vi "Other Output Item UI Update.vi"(8 "error in (no error)":errorcluster, 10 "Other UI Elements":T1, 11 "Output":T2) -> (0 "error out":errorcluster)   [LabVIEW 2015, in "OutputUI.lvclass"]
uses:
  OutputUI.lvclass
  Step/STEP_OUTPUT.ctl
  Step/OUTPUT_DATA_TYPE.ctl
  OUTPUT_CHECK_TYPE.ctl
  Step/OUTPUT_VALUE_TYPE.ctl
  Step.lvclass
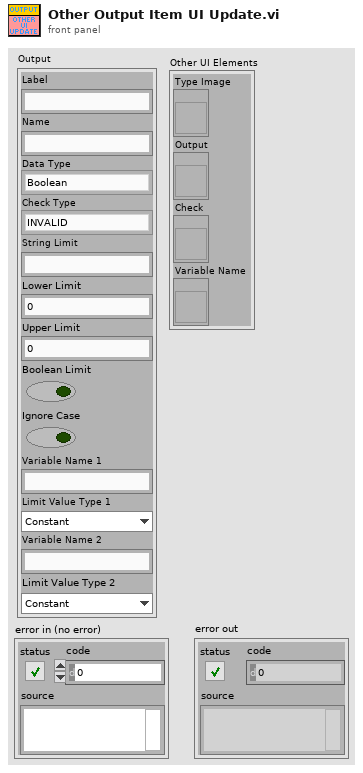
[diagram p1: front panel]
types:
  T1 = cluster{"Type Image":refnum<vi>, "Output":refnum<vi>, "Check":refnum<vi>, "Variable Name":refnum<vi>}
  T2 = typedef "Step.lvclass/STEP_OUTPUT.ctl" = cluster{"Label":string, "Name":string, "Data Type":T3, "Check Type":T4, "String Limit":string, "Lower Limit":dbl, "Upper Limit":dbl, "Boolean Limit":bool, "Ignore Case":bool, "Variable Name 1":string, "Limit Value Type 1":T5, "Variable Name 2":string, "Limit Value Type 2":T5}
  T3 = typedef "Step.lvclass/OUTPUT_DATA_TYPE.ctl" = enum16{"Boolean", "String", "Numeric", "Other"}
  T4 = typedef "Step.lvclass/OUTPUT_CHECK_TYPE.ctl" = enum16{"INVALID", "DO_NOT_CHECK", "RECORD", "VARIABLE", "EQUAL", "NOT_EQUAL", "STR_CONTAINS", "STR_START_WITH", "STR_END_WITH", "STR_REGEX_MATCH", "NUM_GT", "NUM_LT", "NUM_GE", "NUM_LE", "NUM_RANGE", "NUM_RANGE_BDY"}
  T5 = typedef "Step.lvclass/OUTPUT_VALUE_TYPE.ctl" = enum16{"Constant", "Variable"}
  T6 = enum8{"Enabled", "Disabled", "Disabled and Grayed Out"}
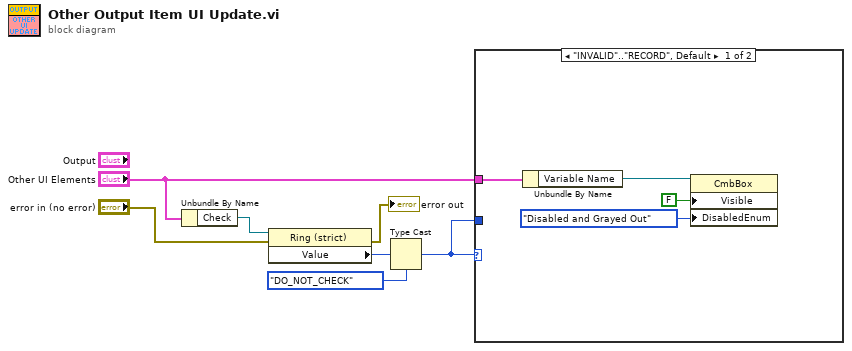
[diagram p0: block diagram]
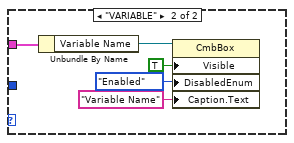
[diagram p2: hidden frame]
diagram:
  n1 = Unbundle By Name("Other UI Elements") -> ("Check"=w7:refnum<vi>)
  n2 = property class="Ring (strict)"(reference=w7, error in="error in (no error)") -> (error out=→"error out":errorcluster, "Value"=w5:u16)  [unwired: 1 out]
  n3 = Type Cast(type=OUTPUT_CHECK_TYPE."DO_NOT_CHECK" ("Check Type"), x=w5) -> (*(type *) &x=w4:T4)
  n4 = case shown="\"INVALID\"..\"RECORD\", Default" w4 {
    tunnel: w4 -> [_ _]
    tunnel: "Other UI Elements" -> [w11 w16]
    frame "INVALID".."RECORD", Default {
      n5 = Unbundle By Name(w11) -> ("Variable Name"=w8:refnum<vi>)
      n6 = property class="CmbBox"(reference=w8, "Visible"=FALSE, "DisabledEnum"=T6."Disabled and Grayed Out" ("Disabled")) -> ()  [unwired: 1 in, 2 out]
    }
    frame "VARIABLE" {
      n7 = Unbundle By Name(w16) -> ("Variable Name"=w13:refnum<vi>)
      n8 = property class="CmbBox"(reference=w13, "Visible"=TRUE, "DisabledEnum"=T6."Enabled" ("Disabled"), "Caption.Text"="Variable Name" ("format string")) -> ()  [unwired: 1 in, 2 out]
    }
  }
